vi "App - analyze RUS V6.vi"() -> ()   [LabVIEW 2015] (continued)
path"=path "D:/Data/Ultrasound/LSCO/LSCO22__130814c/5_Cooling_2nd_try/September_2014/091614/137.30000K_500_2500_2.10000V_0.00000T_Sep16-2014__18-33-45_001_091614.bin", "last mod"=timestamp(3493751625 s since 1904-01-01), "file name str"="D:\\Data\\Ultrasound\\LSCO\\LSCO22__130814c\\5_Cooling_2nd_try\\September_2014\\091614\\137.30000K_500_2500_2.10000V_0.00000T_Sep16-2014__18-33-45_001_091614.bin", "mod time(min)"=58229193.75, "file format"=enum."binary", "power(V)"=2.1, "Magn Field(T) "=0.0}, {"temperature"=137.004, "temperature str"="137.00400", "file path"=path "D:/Data/Ultrasound/LSCO/LSCO22__130814c/5_Cooling_2nd_try/September_2014/091614/137.00400K_500_2500_2.10000V_0.00000T_Sep16-2014__18-35-05_001_091614.bin", "last mod"=timestamp(3493751705 s since 1904-01-01), "file name str"="D:\\Data\\Ultrasound\\LSCO\\LSCO22__130814c\\5_Cooling_2nd_try\\September_2014\\091614\\137.00400K_500_2500_2.10000V_0.00000T_Sep16-2014__18-35-05_001_091614.bin", "mod time(min)"=58229195.083333336, "file format"=enum."binary", "power(V)"=2.1, "Magn Field(T) "=0.0}, {"temperature"=136.689, "temperature str"="136.68900", "file path"=path "D:/Data/Ultrasound/LSCO/LSCO22__130814c/5_Cooling_2nd_try/September_2014/091614/136.68900K_500_2500_2.10000V_0.00000T_Sep16-2014__18-36-24_001_091614.bin", "last mod"=timestamp(3493751784 s since 1904-01-01), "file name str"="D:\\Data\\Ultrasound\\LSCO\\LSCO22__130814c\\5_Cooling_2nd_try\\September_2014\\091614\\136.68900K_500_2500_2.10000V_0.00000T_Sep16-2014__18-36-24_001_091614.bin", "mod time(min)"=58229196.4, "file format"=enum."binary", "power(V)"=2.1, "Magn Field(T) "=0.0}, {"temperature"=136.379, "temperature str"="136.37900", "file path"=path "D:/Data/Ultrasound/LSCO/LSCO22__130814c/5_Cooling_2nd_try/September_2014/091614/136.37900K_500_2500_2.10000V_0.00000T_Sep16-2014__18-37-44_001_091614.bin", "last mod"=timestamp(3493751864 s since 1904-01-01), "file name str"="D:\\Data\\Ultrasound\\LSCO\\LSCO22__130814c\\5_Cooling_2nd_try\\September_2014\\091614\\136.37900K_500_2500_2.10000V_0.00000T_Sep16-2014__18-37-44_001_091614.bin", "mod time(min)"=58229197.733333334, "file format"=enum."binary", "power(V)"=2.1, "Magn Field(T) "=0.0}, {"temperature"=136.08, "temperature str"="136.08000", "file path"=path "D:/Data/Ultrasound/LSCO/LSCO22__130814c/5_Cooling_2nd_try/September_2014/091614/136.08000K_500_2500_2.10000V_0.00000T_Sep16-2014__18-39-03_001_091614.bin", "last mod"=timestamp(3493751943 s since 1904-01-01), "file name str"="D:\\Data\\Ultrasound\\LSCO\\LSCO22__130814c\\5_Cooling_2nd_try\\September_2014\\091614\\136.08000K_500_2500_2.10000V_0.00000T_Sep16-2014__18-39-03_001_091614.bin", "mod time(min)"=58229199.05, "file format"=enum."binary", "power(V)"=2.1, "Magn Field(T) "=0.0}, {"temperature"=135.77, "temperature str"="135.77000", "file path"=path "D:/Data/Ultrasound/LSCO/LSCO22__130814c/5_Cooling_2nd_try/September_2014/091614/135.77000K_500_2500_2.10000V_0.00000T_Sep16-2014__18-40-22_001_091614.bin", "last mod"=timestamp(3493752022 s since 1904-01-01), "file name str"="D:\\Data\\Ultrasound\\LSCO\\LSCO22__130814c\\5_Cooling_2nd_try\\September_2014\\091614\\135.77000K_500_2500_2.10000V_0.00000T_Sep16-2014__18-40-22_001_091614.bin", "mod time(min)"=58229200.36666667, "file format"=enum."binary", "power(V)"=2.1, "Magn Field(T) "=0.0}, {"temperature"=135.475, "temperature str"="135.47500", "file path"=path "D:/Data/Ultrasound/LSCO/LSCO22__130814c/5_Cooling_2nd_try/September_2014/091614/135.47500K_500_2500_2.10000V_0.00000T_Sep16-2014__18-41-42_001_091614.bin", "last mod"=timestamp(3493752102 s since 1904-01-01), "file name str"="D:\\Data\\Ultrasound\\LSCO\\LSCO22__130814c\\5_Cooling_2nd_try\\September_2014\\091614\\135.47500K_500_2500_2.10000V_0.00000T_Sep16-2014__18-41-42_001_091614.bin", "mod time(min)"=58229201.7, "file format"=enum."binary", "power(V)"=2.1, "Magn Field(T) "=0.0}, {"temperature"=135.167, "temperature str"="135.16700", "file path"=path "D:/Data/Ultrasound/LSCO/LSCO22__130814c/5_Cooling_2nd_try/September_2014/091614/135.16700K_500_2500_2.10000V_0.00000T_Sep16-2014__18-43-01_001_091614.bin", "last mod"=timestamp(3493752181 s since 1904-01-01), "file name str"="D:\\Data\\Ultrasound\\LSCO\\LSCO22__130814c\\5_Cooling_2nd_try\\September_2014\\091614\\135.16700K_500_2500_2.10000V_0.00000T_Sep16-2014__18-43-01_001_091614.bin", "mod time(min)"=58229203.016666666, "file format"=enum."binary", "power(V)"=2.1, "Magn Field(T) "=0.0}, {"temperature"=134.859, "temperature str"="134.85900", "file path"=path "D:/Data/Ultrasound/LSCO/LSCO22__130814c/5_Cooling_2nd_try/September_2014/091614/134.85900K_500_2500_2.10000V_0.00000T_Sep16-2014__18-44-20_001_091614.bin", "last mod"=timestamp(3493752260 s since 1904-01-01), "file name str"="D:\\Data\\Ultrasound\\LSCO\\LSCO22__130814c\\5_Cooling_2nd_try\\September_2014\\091614\\134.85900K_500_2500_2.10000V_0.00000T_Sep16-2014__18-44-20_001_091614.bin", "mod time(min)"=58229204.333333336, "file format"=enum."binary", "power(V)"=2.1, "Magn Field(T) "=0.0}, {"temperature"=134.565, "temperature str"="134.56500", "file path"=path "D:/Data/Ultrasound/LSCO/LSCO22__130814c/5_Cooling_2nd_try/September_2014/091614/134.56500K_500_2500_2.10000V_0.00000T_Sep16-2014__18-45-40_001_091614.bin", "last mod"=timestamp(3493752340 s since 1904-01-01), "file name str"="D:\\Data\\Ultrasound\\LSCO\\LSCO22__130814c\\5_Cooling_2nd_try\\September_2014\\091614\\134.56500K_500_2500_2.10000V_0.00000T_Sep16-2014__18-45-40_001_091614.bin", "mod time(min)"=58229205.666666664, "file format"=enum."binary", "power(V)"=2.1, "Magn Field(T) "=0.0}, {"temperature"=134.259, "temperature str"="134.25900", "file path"=path "D:/Data/Ultrasound/LSCO/LSCO22__130814c/5_Cooling_2nd_try/September_2014/091614/134.25900K_500_2500_2.10000V_0.00000T_Sep16-2014__18-46-59_001_091614.bin", "last mod"=timestamp(3493752419 s since 1904-01-01), "file name str"="D:\\Data\\Ultrasound\\LSCO\\LSCO22__130814c\\5_Cooling_2nd_try\\September_2014\\091614\\134.25900K_500_2500_2.10000V_0.00000T_Sep16-2014__18-46-59_001_091614.bin", "mod time(min)"=58229206.983333334, "file format"=enum."binary", "power(V)"=2.1, "Magn Field(T) "=0.0}, {"temperature"=133.967, "temperature str"="133.96700", "file path"=path "D:/Data/Ultrasound/LSCO/LSCO22__130814c/5_Cooling_2nd_try/September_2014/091614/133.96700K_500_2500_2.10000V_0.00000T_Sep16-2014__18-48-19_001_091614.bin", "last mod"=timestamp(3493752499 s since 1904-01-01), "file name str"="D:\\Data\\Ultrasound\\LSCO\\LSCO22__130814c\\5_Cooling_2nd_try\\September_2014\\091614\\133.96700K_500_2500_2.10000V_0.00000T_Sep16-2014__18-48-19_001_091614.bin", "mod time(min)"=58229208.31666667, "file format"=enum."binary", "power(V)"=2.1, "Magn Field(T) "=0.0}, {"temperature"=133.655, "temperature str"="133.65500", "file path"=path "D:/Data/Ultrasound/LSCO/LSCO22__130814c/5_Cooling_2nd_try/September_2014/091614/133.65500K_500_2500_2.10000V_0.00000T_Sep16-2014__18-49-38_001_091614.bin", "last mod"=timestamp(3493752578 s since 1904-01-01), "file name str"="D:\\Data\\Ultrasound\\LSCO\\LSCO22__130814c\\5_Cooling_2nd_try\\September_2014\\091614\\133.65500K_500_2500_2.10000V_0.00000T_Sep16-2014__18-49-38_001_091614.bin", "mod time(min)"=58229209.63333333, "file format"=enum."binary", "power(V)"=2.1, "Magn Field(T) "=0.0}, {"temperature"=133.359, "temperature str"="133.35900", "file path"=path "D:/Data/Ultrasound/LSCO/LSCO22__130814c/5_Cooling_2nd_try/September_2014/091614/133.35900K_500_2500_2.10000V_0.00000T_Sep16-2014__18-50-57_001_091614.bin", "last mod"=timestamp(3493752657 s since 1904-01-01), "file name str"="D:\\Data\\Ultrasound\\LSCO\\LSCO22__130814c\\5_Cooling_2nd_try\\September_2014\\091614\\133.35900K_500_2500_2.10000V_0.00000T_Sep16-2014__18-50-57_001_091614.bin", "mod time(min)"=58229210.95, "file format"=enum."binary", "power(V)"=2.1, "Magn Field(T) "=0.0}, {"temperature"=133.076, "temperature str"="133.07600", "file path"=path "D:/Data/Ultrasound/LSCO/LSCO22__130814c/5_Cooling_2nd_try/September_2014/091614/133.07600K_500_2500_2.10000V_0.00000T_Sep16-2014__18-52-17_001_091614.bin", "last mod"=timestamp(3493752737 s since 1904-01-01), "file name str"="D:\\Data\\Ultrasound\\LSCO\\LSCO22__130814c\\5_Cooling_2nd_try\\September_2014\\091614\\133.07600K_500_2500_2.10000V_0.00000T_Sep16-2014__18-52-17_001_091614.bin", "mod time(min)"=58229212.28333333, "file format"=enum."binary", "power(V)"=2.1, "Magn Field(T) "=0.0}, {"temperature"=132.767, "temperature str"="132.76700", "file path"=path "D:/Data/Ultrasound/LSCO/LSCO22__130814c/5_Cooling_2nd_try/September_2014/091614/132.76700K_500_2500_2.10000V_0.00000T_Sep16-2014__18-53-36_001_091614.bin", "last mod"=timestamp(3493752816 s since 1904-01-01), "file name str"="D:\\Data\\Ultrasound\\LSCO\\LSCO22__130814c\\5_Cooling_2nd_try\\September_2014\\091614\\132.76700K_500_2500_2.10000V_0.00000T_Sep16-2014__18-53-36_001_091614.bin", "mod time(min)"=58229213.6, "file format"=enum."binary", "power(V)"=2.1, "Magn Field(T) "=0.0}, {"temperature"=132.465, "temperature str"="132.46500", "file path"=path "D:/Data/Ultrasound/LSCO/LSCO22__130814c/5_Cooling_2nd_try/September_2014/091614/132.46500K_500_2500_2.10000V_0.00000T_Sep16-2014__18-54-56_001_091614.bin", "last mod"=timestamp(3493752896 s since 1904-01-01), "file name str"="D:\\Data\\Ultrasound\\LSCO\\LSCO22__130814c\\5_Cooling_2nd_try\\September_2014\\091614\\132.46500K_500_2500_2.10000V_0.00000T_Sep16-2014__18-54-56_001_091614.bin", "mod time(min)"=58229214.93333333, "file format"=enum."binary", "power(V)"=2.1, "Magn Field(T) "=0.0}, {"temperature"=132.185, "temperature str"="132.18500", "file path"=path "D:/Data/Ultrasound/LSCO/LSCO22__130814c/5_Cooling_2nd_try/September_2014/091614/132.18500K_500_2500_2.10000V_0.00000T_Sep16-2014__18-56-15_001_091614.bin", "last mod"=timestamp(3493752975 s since 1904-01-01), "file name str"="D:\\Data\\Ultrasound\\LSCO\\LSCO22__130814c\\5_Cooling_2nd_try\\September_2014\\091614\\132.18500K_500_2500_2.10000V_0.00000T_Sep16-2014__18-56-15_001_091614.bin", "mod time(min)"=58229216.25, "file format"=enum."binary", "power(V)"=2.1, "Magn Field(T) "=0.0}, {"temperature"=131.882, "temperature str"="131.88200", "file path"=path "D:/Data/Ultrasound/LSCO/LSCO22__130814c/5_Cooling_2nd_try/September_2014/091614/131.88200K_500_2500_2.10000V_0.00000T_Sep16-2014__18-57-34_001_091614.bin", "last mod"=timestamp(3493753054 s since 1904-01-01), "file name str"="D:\\Data\\Ultrasound\\LSCO\\LSCO22__130814c\\5_Cooling_2nd_try\\September_2014\\091614\\131.88200K_500_2500_2.10000V_0.00000T_Sep16-2014__18-57-34_001_091614.bin", "mod time(min)"=58229217.56666667, "file format"=enum."binary", "power(V)"=2.1, "Magn Field(T) "=0.0}, {"temperature"=131.592, "temperature str"="131.59200", "file path"=path "D:/Data/Ultrasound/LSCO/LSCO22__130814c/5_Cooling_2nd_try/September_2014/091614/131.59200K_500_2500_2.10000V_0.00000T_Sep16-2014__18-58-54_001_091614.bin", "last mod"=timestamp(3493753134 s since 1904-01-01), "file name str"="D:\\Data\\Ultrasound\\LSCO\\LSCO22__130814c\\5_Cooling_2nd_try\\September_2014\\091614\\131.59200K_500_2500_2.10000V_0.00000T_Sep16-2014__18-58-54_001_091614.bin", "mod time(min)"=58229218.9, "file format"=enum."binary", "power(V)"=2.1, "Magn Field(T) "=0.0}, {"temperature"=131.299, "temperature str"="131.29900", "file path"=path "D:/Data/Ultrasound/LSCO/LSCO22__130814c/5_Cooling_2nd_try/September_2014/091614/131.29900K_500_2500_2.10000V_0.00000T_Sep16-2014__19-00-13_001_091614.bin", "last mod"=timestamp(3493753213 s since 1904-01-01), "file name str"="D:\\Data\\Ultrasound\\LSCO\\LSCO22__130814c\\5_Cooling_2nd_try\\September_2014\\091614\\131.29900K_500_2500_2.10000V_0.00000T_Sep16-2014__19-00-13_001_091614.bin", "mod time(min)"=58229220.21666667, "file format"=enum."binary", "power(V)"=2.1, "Magn Field(T) "=0.0}, {"temperature"=131.007, "temperature str"="131.00700", "file path"=path "D:/Data/Ultrasound/LSCO/LSCO22__130814c/5_Cooling_2nd_try/September_2014/091614/131.00700K_500_2500_2.10000V_0.00000T_Sep16-2014__19-01-32_001_091614.bin", "last mod"=timestamp(3493753292 s since 1904-01-01), "file name str"="D:\\Data\\Ultrasound\\LSCO\\LSCO22__130814c\\5_Cooling_2nd_try\\September_2014\\091614\\131.00700K_500_2500_2.10000V_0.00000T_Sep16-2014__19-01-32_001_091614.bin", "mod time(min)"=58229221.53333333, "file format"=enum."binary", "power(V)"=2.1, "Magn Field(T) "=0.0}, {"temperature"=130.718, "temperature str"="130.71800", "file path"=path "D:/Data/Ultrasound/LSCO/LSCO22__130814c/5_Cooling_2nd_try/September_2014/091614/130.71800K_500_2500_2.10000V_0.00000T_Sep16-2014__19-02-52_001_091614.bin", "last mod"=timestamp(3493753372 s since 1904-01-01), "file name str"="D:\\Data\\Ultrasound\\LSCO\\LSCO22__130814c\\5_Cooling_2nd_try\\September_2014\\091614\\130.71800K_500_2500_2.10000V_0.00000T_Sep16-2014__19-02-52_001_091614.bin", "mod time(min)"=58229222.86666667, "file format"=enum."binary", "power(V)"=2.1, "Magn Field(T) "=0.0}, {"temperature"=130.427, "temperature str"="130.42700", "file path"=path "D:/Data/Ultrasound/LSCO/LSCO22__130814c/5_Cooling_2nd_try/September_2014/091614/130.42700K_500_2500_2.10000V_0.00000T_Sep16-2014__19-04-11_001_091614.bin", "last mod"=timestamp(3493753451 s since 1904-01-01), "file name str"="D:\\Data\\Ultrasound\\LSCO\\LSCO22__130814c\\5_Cooling_2nd_try\\September_2014\\091614\\130.42700K_500_2500_2.10000V_0.00000T_Sep16-2014__19-04-11_001_091614.bin", "mod time(min)"=58229224.18333333, "file format"=enum."binary", "power(V)"=2.1, "Magn Field(T) "=0.0}, {"temperature"=130.147, "temperature str"="130.14700", "file path"=path "D:/Data/Ultrasound/LSCO/LSCO22__130814c/5_Cooling_2nd_try/September_2014/091614/130.14700K_500_2500_2.10000V_0.00000T_Sep16-2014__19-05-31_001_091614.bin", "last mod"=timestamp(3493753531 s since 1904-01-01), "file name str"="D:\\Data\\Ultrasound\\LSCO\\LSCO22__130814c\\5_Cooling_2nd_try\\September_2014\\091614\\130.14700K_500_2500_2.10000V_0.00000T_Sep16-2014__19-05-31_001_091614.bin", "mod time(min)"=58229225.516666666, "file format"=enum."binary", "power(V)"=2.1, "Magn Field(T) "=0.0}, {"temperature"=129.849, "temperature str"="129.84900", "file path"=path "D:/Data/Ultrasound/LSCO/LSCO22__130814c/5_Cooling_2nd_try/September_2014/091614/129.84900K_500_2500_2.10000V_0.00000T_Sep16-2014__19-06-50_001_091614.bin", "last mod"=timestamp(3493753610 s since 1904-01-01), "file name str"="D:\\Data\\Ultrasound\\LSCO\\LSCO22__130814c\\5_Cooling_2nd_try\\September_2014\\091614\\129.84900K_500_2500_2.10000V_0.00000T_Sep16-2014__19-06-50_001_091614.bin", "mod time(min)"=58229226.833333336, "file format"=enum."binary", "power(V)"=2.1, "Magn Field(T) "=0.0}, {"temperature"=129.561, "temperature str"="129.56100", "file path"=path "D:/Data/Ultrasound/LSCO/LSCO22__130814c/5_Cooling_2nd_try/September_2014/091614/129.56100K_500_2500_2.10000V_0.00000T_Sep16-2014__19-08-09_001_091614.bin", "last mod"=timestamp(3493753689 s since 1904-01-01), "file name str"="D:\\Data\\Ultrasound\\LSCO\\LSCO22__130814c\\5_Cooling_2nd_try\\September_2014\\091614\\129.56100K_500_2500_2.10000V_0.00000T_Sep16-2014__19-08-09_001_091614.bin", "mod time(min)"=58229228.15, "file format"=enum."binary", "power(V)"=2.1, "Magn Field(T) "=0.0}, {"temperature"=129.282, "temperature str"="129.28200", "file path"=path "D:/Data/Ultrasound/LSCO/LSCO22__130814c/5_Cooling_2nd_try/September_2014/091614/129.28200K_500_2500_2.10000V_0.00000T_Sep16-2014__19-09-29_001_091614.bin", "last mod"=timestamp(3493753769 s since 1904-01-01), "file name str"="D:\\Data\\Ultrasound\\LSCO\\LSCO22__130814c\\5_Cooling_2nd_try\\September_2014\\091614\\129.28200K_500_2500_2.10000V_0.00000T_Sep16-2014__19-09-29_001_091614.bin", "mod time(min)"=58229229.483333334, "file format"=enum."binary", "power(V)"=2.1, "Magn Field(T) "=0.0}, {"temperature"=128.991, "temperature str"="128.99100", "file path"=path "D:/Data/Ultrasound/LSCO/LSCO22__130814c/5_Cooling_2nd_try/September_2014/091614/128.99100K_500_2500_2.10000V_0.00000T_Sep16-2014__19-10-48_001_091614.bin", "last mod"=timestamp(3493753848 s since 1904-01-01), "file name str"="D:\\Data\\Ultrasound\\LSCO\\LSCO22__130814c\\5_Cooling_2nd_try\\September_2014\\091614\\128.99100K_500_2500_2.10000V_0.00000T_Sep16-2014__19-10-48_001_091614.bin", "mod time(min)"=58229230.8, "file format"=enum."binary", "power(V)"=2.1, "Magn Field(T) "=0.0}, {"temperature"=128.717, "temperature str"="128.71700", "file path"=path "D:/Data/Ultrasound/LSCO/LSCO22__130814c/5_Cooling_2nd_try/September_2014/091614/128.71700K_500_2500_2.10000V_0.00000T_Sep16-2014__19-12-07_001_091614.bin", "last mod"=timestamp(3493753927 s since 1904-01-01), "file name str"="D:\\Data\\Ultrasound\\LSCO\\LSCO22__130814c\\5_Cooling_2nd_try\\September_2014\\091614\\128.71700K_500_2500_2.10000V_0.00000T_Sep16-2014__19-12-07_001_091614.bin", "mod time(min)"=58229232.11666667, "file format"=enum."binary", "power(V)"=2.1, "Magn Field(T) "=0.0}, {"temperature"=128.421, "temperature str"="128.42100", "file path"=path "D:/Data/Ultrasound/LSCO/LSCO22__130814c/5_Cooling_2nd_try/September_2014/091614/128.42100K_500_2500_2.10000V_0.00000T_Sep16-2014__19-13-27_001_091614.bin", "last mod"=timestamp(3493754007 s since 1904-01-01), "file name str"="D:\\Data\\Ultrasound\\LSCO\\LSCO22__130814c\\5_Cooling_2nd_try\\September_2014\\091614\\128.42100K_500_2500_2.10000V_0.00000T_Sep16-2014__19-13-27_001_091614.bin", "mod time(min)"=58229233.45, "file format"=enum."binary", "power(V)"=2.1, "Magn Field(T) "=0.0}, {"temperature"=128.135, "temperature str"="128.13500", "file path"=path "D:/Data/Ultrasound/LSCO/LSCO22__130814c/5_Cooling_2nd_try/September_2014/091614/128.13500K_500_2500_2.10000V_0.00000T_Sep16-2014__19-14-46_001_091614.bin", "last mod"=timestamp(3493754086 s since 1904-01-01), "file name str"="D:\\Data\\Ultrasound\\LSCO\\LSCO22__130814c\\5_Cooling_2nd_try\\September_2014\\091614\\128.13500K_500_2500_2.10000V_0.00000T_Sep16-2014__19-14-46_001_091614.bin", "mod time(min)"=58229234.766666666, "file format"=enum."binary", "power(V)"=2.1, "Magn Field(T) "=0.0}, {"temperature"=127.874, "temperature str"="127.87400", "file path"=path "D:/Data/Ultrasound/LSCO/LSCO22__130814c/5_Cooling_2nd_try/September_2014/091614/127.87400K_500_2500_2.10000V_0.00000T_Sep16-2014__19-16-06_001_091614.bin", "last mod"=timestamp(3493754166 s since 1904-01-01), "file name str"="D:\\Data\\Ultrasound\\LSCO\\LSCO22__130814c\\5_Cooling_2nd_try\\September_2014\\091614\\127.87400K_500_2500_2.10000V_0.00000T_Sep16-2014__19-16-06_001_091614.bin", "mod time(min)"=58229236.1, "file format"=enum."binary", "power(V)"=2.1, "Magn Field(T) "=0.0}, {"temperature"=127.58, "temperature str"="127.58000", "file path"=path "D:/Data/Ultrasound/LSCO/LSCO22__130814c/5_Cooling_2nd_try/September_2014/091614/127.58000K_500_2500_2.10000V_0.00000T_Sep16-2014__19-17-25_001_091614.bin", "last mod"=timestamp(3493754245 s since 1904-01-01), "file name str"="D:\\Data\\Ultrasound\\LSCO\\LSCO22__130814c\\5_Cooling_2nd_try\\September_2014\\091614\\127.58000K_500_2500_2.10000V_0.00000T_Sep16-2014__19-17-25_001_091614.bin", "mod time(min)"=58229237.416666664, "file format"=enum."binary", "power(V)"=2.1, "Magn Field(T) "=0.0}, {"temperature"=127.303, "temperature str"="127.30300", "file path"=path "D:/Data/Ultrasound/LSCO/LSCO22__130814c/5_Cooling_2nd_try/September_2014/091614/127.30300K_500_2500_2.10000V_0.00000T_Sep16-2014__19-18-44_001_091614.bin", "last mod"=timestamp(3493754324 s since 1904-01-01), "file name str"="D:\\Data\\Ultrasound\\LSCO\\LSCO22__130814c\\5_Cooling_2nd_try\\September_2014\\091614\\127.30300K_500_2500_2.10000V_0.00000T_Sep16-2014__19-18-44_001_091614.bin", "mod time(min)"=58229238.733333334, "file format"=enum."binary", "power(V)"=2.1, "Magn Field(T) "=0.0}, {"temperature"=127.032, "temperature str"="127.03200", "file path"=path "D:/Data/Ultrasound/LSCO/LSCO22__130814c/5_Cooling_2nd_try/September_2014/091614/127.03200K_500_2500_2.10000V_0.00000T_Sep16-2014__19-20-04_001_091614.bin", "last mod"=timestamp(3493754404 s since 1904-01-01), "file name str"="D:\\Data\\Ultrasound\\LSCO\\LSCO22__130814c\\5_Cooling_2nd_try\\September_2014\\091614\\127.03200K_500_2500_2.10000V_0.00000T_Sep16-2014__19-20-04_001_091614.bin", "mod time(min)"=58229240.06666667, "file format"=enum."binary", "power(V)"=2.1, "Magn Field(T) "=0.0}, {"temperature"=126.745, "temperature str"="126.74500", "file path"=path "D:/Data/Ultrasound/LSCO/LSCO22__130814c/5_Cooling_2nd_try/September_2014/091614/126.74500K_500_2500_2.10000V_0.00000T_Sep16-2014__19-21-23_001_091614.bin", "last mod"=timestamp(3493754483 s since 1904-01-01), "file name str"="D:\\Data\\Ultrasound\\LSCO\\LSCO22__130814c\\5_Cooling_2nd_try\\September_2014\\091614\\126.74500K_500_2500_2.10000V_0.00000T_Sep16-2014__19-21-23_001_091614.bin", "mod time(min)"=58229241.38333333, "file format"=enum."binary", "power(V)"=2.1, "Magn Field(T) "=0.0}, {"temperature"=126.472, "temperature str"="126.47200", "file path"=path "D:/Data/Ultrasound/LSCO/LSCO22__130814c/5_Cooling_2nd_try/September_2014/091614/126.47200K_500_2500_2.10000V_0.00000T_Sep16-2014__19-22-43_001_091614.bin", "last mod"=timestamp(3493754563 s since 1904-01-01), "file name str"="D:\\Data\\Ultrasound\\LSCO\\LSCO22__130814c\\5_Cooling_2nd_try\\September_2014\\091614\\126.47200K_500_2500_2.10000V_0.00000T_Sep16-2014__19-22-43_001_091614.bin", "mod time(min)"=58229242.71666667, "file format"=enum."binary", "power(V)"=2.1, "Magn Field(T) "=0.0}, {"temperature"=126.195, "temperature str"="126.19500", "file path"=path "D:/Data/Ultrasound/LSCO/LSCO22__130814c/5_Cooling_2nd_try/September_2014/091614/126.19500K_500_2500_2.10000V_0.00000T_Sep16-2014__19-24-02_001_091614.bin", "last mod"=timestamp(3493754642 s since 1904-01-01), "file name str"="D:\\Data\\Ultrasound\\LSCO\\LSCO22__130814c\\5_Cooling_2nd_try\\September_2014\\091614\\126.19500K_500_2500_2.10000V_0.00000T_Sep16-2014__19-24-02_001_091614.bin", "mod time(min)"=58229244.03333333, "file format"=enum."binary", "power(V)"=2.1, "Magn Field(T) "=0.0}, {"temperature"=125.926, "temperature str"="125.92600", "file path"=path "D:/Data/Ultrasound/LSCO/LSCO22__130814c/5_Cooling_2nd_try/September_2014/091614/125.92600K_500_2500_2.10000V_0.00000T_Sep16-2014__19-25-21_001_091614.bin", "last mod"=timestamp(3493754721 s since 1904-01-01), "file name str"="D:\\Data\\Ultrasound\\LSCO\\LSCO22__130814c\\5_Cooling_2nd_try\\September_2014\\091614\\125.92600K_500_2500_2.10000V_0.00000T_Sep16-2014__19-25-21_001_091614.bin", "mod time(min)"=58229245.35, "file format"=enum."binary", "power(V)"=2.1, "Magn Field(T) "=0.0}, {"temperature"=125.648, "temperature str"="125.64800", "file path"=path "D:/Data/Ultrasound/LSCO/LSCO22__130814c/5_Cooling_2nd_try/September_2014/091614/125.64800K_500_2500_2.10000V_0.00000T_Sep16-2014__19-26-41_001_091614.bin", "last mod"=timestamp(3493754801 s since 1904-01-01), "file name str"="D:\\Data\\Ultrasound\\LSCO\\LSCO22__130814c\\5_Cooling_2nd_try\\September_2014\\091614\\125.64800K_500_2500_2.10000V_0.00000T_Sep16-2014__19-26-41_001_091614.bin", "mod time(min)"=58229246.68333333, "file format"=enum."binary", "power(V)"=2.1, "Magn Field(T) "=0.0}, {"temperature"=125.371, "temperature str"="125.37100", "file path"=path "D:/Data/Ultrasound/LSCO/LSCO22__130814c/5_Cooling_2nd_try/September_2014/091614/125.37100K_500_2500_2.10000V_0.00000T_Sep16-2014__19-28-00_001_091614.bin", "last mod"=timestamp(3493754880 s since 1904-01-01), "file name str"="D:\\Data\\Ultrasound\\LSCO\\LSCO22__130814c\\5_Cooling_2nd_try\\September_2014\\091614\\125.37100K_500_2500_2.10000V_0.00000T_Sep16-2014__19-28-00_001_091614.bin", "mod time(min)"=58229248.0, "file format"=enum."binary", "power(V)"=2.1, "Magn Field(T) "=0.0}, {"temperature"=125.102, "temperature str"="125.10200", "file path"=path "D:/Data/Ultrasound/LSCO/LSCO22__130814c/5_Cooling_2nd_try/September_2014/091614/125.10200K_500_2500_2.10000V_0.00000T_Sep16-2014__19-29-19_001_091614.bin", "last mod"=timestamp(3493754959 s since 1904-01-01), "file name str"="D:\\Data\\Ultrasound\\LSCO\\LSCO22__130814c\\5_Cooling_2nd_try\\September_2014\\091614\\125.10200K_500_2500_2.10000V_0.00000T_Sep16-2014__19-29-19_001_091614.bin", "mod time(min)"=58229249.31666667, "file format"=enum."binary", "power(V)"=2.1, "Magn Field(T) "=0.0}, {"temperature"=124.83, "temperature str"="124.83000", "file path"=path "D:/Data/Ultrasound/LSCO/LSCO22__130814c/5_Cooling_2nd_try/September_2014/091614/124.83000K_500_2500_2.10000V_0.00000T_Sep16-2014__19-30-39_001_091614.bin", "last mod"=timestamp(3493755039 s since 1904-01-01), "file name str"="D:\\Data\\Ultrasound\\LSCO\\LSCO22__130814c\\5_Cooling_2nd_try\\September_2014\\091614\\124.83000K_500_2500_2.10000V_0.00000T_Sep16-2014__19-30-39_001_091614.bin", "mod time(min)"=58229250.65, "file format"=enum."binary", "power(V)"=2.1, "Magn Field(T) "=0.0}, {"temperature"=124.565, "temperature str"="124.56500", "file path"=path "D:/Data/Ultrasound/LSCO/LSCO22__130814c/5_Cooling_2nd_try/September_2014/091614/124.56500K_500_2500_2.10000V_0.00000T_Sep16-2014__19-31-58_001_091614.bin", "last mod"=timestamp(3493755118 s since 1904-01-01), "file name str"="D:\\Data\\Ultrasound\\LSCO\\LSCO22__130814c\\5_Cooling_2nd_try\\September_2014\\091614\\124.56500K_500_2500_2.10000V_0.00000T_Sep16-2014__19-31-58_001_091614.bin", "mod time(min)"=58229251.96666667, "file format"=enum."binary", "power(V)"=2.1, "Magn Field(T) "=0.0}, {"temperature"=124.29, "temperature str"="124.29000", "file path"=path "D:/Data/Ultrasound/LSCO/LSCO22__130814c/5_Cooling_2nd_try/September_2014/091614/124.29000K_500_2500_2.10000V_0.00000T_Sep16-2014__19-33-18_001_091614.bin", "last mod"=timestamp(3493755198 s since 1904-01-01), "file name str"="D:\\Data\\Ultrasound\\LSCO\\LSCO22__130814c\\5_Cooling_2nd_try\\September_2014\\091614\\124.29000K_500_2500_2.10000V_0.00000T_Sep16-2014__19-33-18_001_091614.bin", "mod time(min)"=58229253.3, "file format"=enum."binary", "power(V)"=2.1, "Magn Field(T) "=0.0}, {"temperature"=124.019, "temperature str"="124.01900", "file path"=path "D:/Data/Ultrasound/LSCO/LSCO22__130814c/5_Cooling_2nd_try/September_2014/091614/124.01900K_500_2500_2.10000V_0.00000T_Sep16-2014__19-34-37_001_091614.bin", "last mod"=timestamp(3493755277 s since 1904-01-01), "file name str"="D:\\Data\\Ultrasound\\LSCO\\LSCO22__130814c\\5_Cooling_2nd_try\\September_2014\\091614\\124.01900K_500_2500_2.10000V_0.00000T_Sep16-2014__19-34-37_001_091614.bin", "mod time(min)"=58229254.61666667, "file format"=enum."binary", "power(V)"=2.1, "Magn Field(T) "=0.0}, {"temperature"=123.76, "temperature str"="123.76000", "file path"=path "D:/Data/Ultrasound/LSCO/LSCO22__130814c/5_Cooling_2nd_try/September_2014/091614/123.76000K_500_2500_2.10000V_0.00000T_Sep16-2014__19-35-56_001_091614.bin", "last mod"=timestamp(3493755356 s since 1904-01-01), "file name str"="D:\\Data\\Ultrasound\\LSCO\\LSCO22__130814c\\5_Cooling_2nd_try\\September_2014\\091614\\123.76000K_500_2500_2.10000V_0.00000T_Sep16-2014__19-35-56_001_091614.bin", "mod time(min)"=58229255.93333333, "file format"=enum."binary", "power(V)"=2.1, "Magn Field(T) "=0.0}, {"temperature"=123.485, "temperature str"="123.48500", "file path"=path "D:/Data/Ultrasound/LSCO/LSCO22__130814c/5_Cooling_2nd_try/September_2014/091614/123.48500K_500_2500_2.10000V_0.00000T_Sep16-2014__19-37-16_001_091614.bin", "last mod"=timestamp(3493755436 s since 1904-01-01), "file name str"="D:\\Data\\Ultrasound\\LSCO\\LSCO22__130814c\\5_Cooling_2nd_try\\September_2014\\091614\\123.48500K_500_2500_2.10000V_0.00000T_Sep16-2014__19-37-16_001_091614.bin", "mod time(min)"=58229257.266666666, "file format"=enum."binary", "power(V)"=2.1, "Magn Field(T) "=0.0}, {"temperature"=123.221, "temperature str"="123.22100", "file path"=path "D:/Data/Ultrasound/LSCO/LSCO22__130814c/5_Cooling_2nd_try/September_2014/091614/123.22100K_500_2500_2.10000V_0.00000T_Sep16-2014__19-38-35_001_091614.bin", "last mod"=timestamp(3493755515 s since 1904-01-01), "file name str"="D:\\Data\\Ultrasound\\LSCO\\LSCO22__130814c\\5_Cooling_2nd_try\\September_2014\\091614\\123.22100K_500_2500_2.10000V_0.00000T_Sep16-2014__19-38-35_001_091614.bin", "mod time(min)"=58229258.583333336, "file format"=enum."binary", "power(V)"=2.1, "Magn Field(T) "=0.0}, {"temperature"=122.957, "temperature str"="122.95700", "file path"=path "D:/Data/Ultrasound/LSCO/LSCO22__130814c/5_Cooling_2nd_try/September_2014/091614/122.95700K_500_2500_2.10000V_0.00000T_Sep16-2014__19-39-54_001_091614.bin", "last mod"=timestamp(3493755594 s since 1904-01-01), "file name str"="D:\\Data\\Ultrasound\\LSCO\\LSCO22__130814c\\5_Cooling_2nd_try\\September_2014\\091614\\122.95700K_500_2500_2.10000V_0.00000T_Sep16-2014__19-39-54_001_091614.bin", "mod time(min)"=58229259.9, "file format"=enum."binary", "power(V)"=2.1, "Magn Field(T) "=0.0}, {"temperature"=122.69, "temperature str"="122.69000", "file path"=path "D:/Data/Ultrasound/LSCO/LSCO22__130814c/5_Cooling_2nd_try/September_2014/091614/122.69000K_500_2500_2.10000V_0.00000T_Sep16-2014__19-41-14_001_091614.bin", "last mod"=timestamp(3493755674 s since 1904-01-01), "file name str"="D:\\Data\\Ultrasound\\LSCO\\LSCO22__130814c\\5_Cooling_2nd_try\\September_2014\\091614\\122.69000K_500_2500_2.10000V_0.00000T_Sep16-2014__19-41-14_001_091614.bin", "mod time(min)"=58229261.233333334, "file format"=enum."binary", "power(V)"=2.1, "Magn Field(T) "=0.0}, {"temperature"=122.431, "temperature str"="122.43100", "file path"=path "D:/Data/Ultrasound/LSCO/LSCO22__130814c/5_Cooling_2nd_try/September_2014/091614/122.43100K_500_2500_2.10000V_0.00000T_Sep16-2014__19-42-33_001_091614.bin", "last mod"=timestamp(3493755753 s since 1904-01-01), "file name str"="D:\\Data\\Ultrasound\\LSCO\\LSCO22__130814c\\5_Cooling_2nd_try\\September_2014\\091614\\122.43100K_500_2500_2.10000V_0.00000T_Sep16-2014__19-42-33_001_091614.bin", "mod time(min)"=58229262.55, "file format"=enum."binary", "power(V)"=2.1, "Magn Field(T) "=0.0}, {"temperature"=122.165, "temperature str"="122.16500", "file path"=path "D:/Data/Ultrasound/LSCO/LSCO22__130814c/5_Cooling_2nd_try/September_2014/091614/122.16500K_500_2500_2.10000V_0.00000T_Sep16-2014__19-43-53_001_091614.bin", "last mod"=timestamp(3493755833 s since 1904-01-01), "file name str"="D:\\Data\\Ultrasound\\LSCO\\LSCO22__130814c\\5_Cooling_2nd_try\\September_2014\\091614\\122.16500K_500_2500_2.10000V_0.00000T_Sep16-2014__19-43-53_001_091614.bin", "mod time(min)"=58229263.88333333, "file format"=enum."binary", "power(V)"=2.1, "Magn Field(T) "=0.0}, {"temperature"=121.901, "temperature str"="121.90100", "file path"=path "D:/Data/Ultrasound/LSCO/LSCO22__130814c/5_Cooling_2nd_try/September_2014/091614/121.90100K_500_2500_2.10000V_0.00000T_Sep16-2014__19-45-12_001_091614.bin", "last mod"=timestamp(3493755912 s since 1904-01-01), "file name str"="D:\\Data\\Ultrasound\\LSCO\\LSCO22__130814c\\5_Cooling_2nd_try\\September_2014\\091614\\121.90100K_500_2500_2.10000V_0.00000T_Sep16-2014__19-45-12_001_091614.bin", "mod time(min)"=58229265.2, "file format"=enum."binary", "power(V)"=2.1, "Magn Field(T) "=0.0}, {"temperature"=121.649, "temperature str"="121.64900", "file path"=path "D:/Data/Ultrasound/LSCO/LSCO22__130814c/5_Cooling_2nd_try/September_2014/091614/121.64900K_500_2500_2.10000V_0.00000T_Sep16-2014__19-46-31_001_091614.bin", "last mod"=timestamp(3493755991 s since 1904-01-01), "file name str"="D:\\Data\\Ultrasound\\LSCO\\LSCO22__130814c\\5_Cooling_2nd_try\\September_2014\\091614\\121.64900K_500_2500_2.10000V_0.00000T_Sep16-2014__19-46-31_001_091614.bin", "mod time(min)"=58229266.516666666, "file format"=enum."binary", "power(V)"=2.1, "Magn Field(T) "=0.0}, {"temperature"=121.386, "temperature str"="121.38600", "file path"=path "D:/Data/Ultrasound/LSCO/LSCO22__130814c/5_Cooling_2nd_try/September_2014/091614/121.38600K_500_2500_2.10000V_0.00000T_Sep16-2014__19-47-51_001_091614.bin", "last mod"=timestamp(3493756071 s since 1904-01-01), "file name str"="D:\\Data\\Ultrasound\\LSCO\\LSCO22__130814c\\5_Cooling_2nd_try\\September_2014\\091614\\121.38600K_500_2500_2.10000V_0.00000T_Sep16-2014__19-47-51_001_091614.bin", "mod time(min)"=58229267.85, "file format"=enum."binary", "power(V)"=2.1, "Magn Field(T) "=0.0}, {"temperature"=121.132, "temperature str"="121.13200", "file path"=path "D:/Data/Ultrasound/LSCO/LSCO22__130814c/5_Cooling_2nd_try/September_2014/091614/121.13200K_500_2500_2.10000V_0.00000T_Sep16-2014__19-49-10_001_091614.bin", "last mod"=timestamp(3493756150 s since 1904-01-01), "file name str"="D:\\Data\\Ultrasound\\LSCO\\LSCO22__130814c\\5_Cooling_2nd_try\\September_2014\\091614\\121.13200K_500_2500_2.10000V_0.00000T_Sep16-2014__19-49-10_001_091614.bin", "mod time(min)"=58229269.166666664, "file format"=enum."binary", "power(V)"=2.1, "Magn Field(T) "=0.0}, {"temperature"=120.874, "temperature str"="120.87400", "file path"=path "D:/Data/Ultrasound/LSCO/LSCO22__130814c/5_Cooling_2nd_try/September_2014/091614/120.87400K_500_2500_2.10000V_0.00000T_Sep16-2014__19-50-30_001_091614.bin", "last mod"=timestamp(3493756230 s since 1904-01-01), "file name str"="D:\\Data\\Ultrasound\\LSCO\\LSCO22__130814c\\5_Cooling_2nd_try\\September_2014\\091614\\120.87400K_500_2500_2.10000V_0.00000T_Sep16-2014__19-50-30_001_091614.bin", "mod time(min)"=58229270.5, "file format"=enum."binary", "power(V)"=2.1, "Magn Field(T) "=0.0}, {"temperature"=120.614, "temperature str"="120.61400", "file path"=path "D:/Data/Ultrasound/LSCO/LSCO22__130814c/5_Cooling_2nd_try/September_2014/091614/120.61400K_500_2500_2.10000V_0.00000T_Sep16-2014__19-51-49_001_091614.bin", "last mod"=timestamp(3493756309 s since 1904-01-01), "file name str"="D:\\Data\\Ultrasound\\LSCO\\LSCO22__130814c\\5_Cooling_2nd_try\\September_2014\\091614\\120.61400K_500_2500_2.10000V_0.00000T_Sep16-2014__19-51-49_001_091614.bin", "mod time(min)"=58229271.81666667, "file format"=enum."binary", "power(V)"=2.1, "Magn Field(T) "=0.0}, {"temperature"=120.365, "temperature str"="120.36500", "file path"=path "D:/Data/Ultrasound/LSCO/LSCO22__130814c/5_Cooling_2nd_try/September_2014/091614/120.36500K_500_2500_2.10000V_0.00000T_Sep16-2014__19-53-08_001_091614.bin", "last mod"=timestamp(3493756388 s since 1904-01-01), "file name str"="D:\\Data\\Ultrasound\\LSCO\\LSCO22__130814c\\5_Cooling_2nd_try\\September_2014\\091614\\120.36500K_500_2500_2.10000V_0.00000T_Sep16-2014__19-53-08_001_091614.bin", "mod time(min)"=58229273.13333333, "file format"=enum."binary", "power(V)"=2.1, "Magn Field(T) "=0.0}, {"temperature"=120.108, "temperature str"="120.10800", "file path"=path "D:/Data/Ultrasound/LSCO/LSCO22__130814c/5_Cooling_2nd_try/September_2014/091614/120.10800K_500_2500_2.10000V_0.00000T_Sep16-2014__19-54-28_001_091614.bin", "last mod"=timestamp(3493756468 s since 1904-01-01), "file name str"="D:\\Data\\Ultrasound\\LSCO\\LSCO22__130814c\\5_Cooling_2nd_try\\September_2014\\091614\\120.10800K_500_2500_2.10000V_0.00000T_Sep16-2014__19-54-28_001_091614.bin", "mod time(min)"=58229274.46666667, "file format"=enum."binary", "power(V)"=2.1, "Magn Field(T) "=0.0}, {"temperature"=119.859, "temperature str"="119.85900", "file path"=path "D:/Data/Ultrasound/LSCO/LSCO22__130814c/5_Cooling_2nd_try/September_2014/091614/119.85900K_500_2500_2.10000V_0.00000T_Sep16-2014__19-55-47_001_091614.bin", "last mod"=timestamp(3493756547 s since 1904-01-01), "file name str"="D:\\Data\\Ultrasound\\LSCO\\LSCO22__130814c\\5_Cooling_2nd_try\\September_2014\\091614\\119.85900K_500_2500_2.10000V_0.00000T_Sep16-2014__19-55-47_001_091614.bin", "mod time(min)"=58229275.78333333, "file format"=enum."binary", "power(V)"=2.1, "Magn Field(T) "=0.0}, {"temperature"=119.604, "temperature str"="119.60400", "file path"=path "D:/Data/Ultrasound/LSCO/LSCO22__130814c/5_Cooling_2nd_try/September_2014/091614/119.60400K_500_2500_2.10000V_0.00000T_Sep16-2014__19-57-06_001_091614.bin", "last mod"=timestamp(3493756626 s since 1904-01-01), "file name str"="D:\\Data\\Ultrasound\\LSCO\\LSCO22__130814c\\5_Cooling_2nd_try\\September_2014\\091614\\119.60400K_500_2500_2.10000V_0.00000T_Sep16-2014__19-57-06_001_091614.bin", "mod time(min)"=58229277.1, "file format"=enum."binary", "power(V)"=2.1, "Magn Field(T) "=0.0}, {"temperature"=119.349, "temperature str"="119.34900", "file path"=path "D:/Data/Ultrasound/LSCO/LSCO22__130814c/5_Cooling_2nd_try/September_2014/091614/119.34900K_500_2500_2.10000V_0.00000T_Sep16-2014__19-58-26_001_091614.bin", "last mod"=timestamp(3493756706 s since 1904-01-01), "file name str"="D:\\Data\\Ultrasound\\LSCO\\LSCO22__130814c\\5_Cooling_2nd_try\\September_2014\\091614\\119.34900K_500_2500_2.10000V_0.00000T_Sep16-2014__19-58-26_001_091614.bin", "mod time(min)"=58229278.43333333, "file format"=enum."binary", "power(V)"=2.1, "Magn Field(T) "=0.0}, {"temperature"=119.104, "temperature str"="119.10400", "file path"=path "D:/Data/Ultrasound/LSCO/LSCO22__130814c/5_Cooling_2nd_try/September_2014/091614/119.10400K_500_2500_2.10000V_0.00000T_Sep16-2014__19-59-45_001_091614.bin", "last mod"=timestamp(3493756785 s since 1904-01-01), "file name str"="D:\\Data\\Ultrasound\\LSCO\\LSCO22__130814c\\5_Cooling_2nd_try\\September_2014\\091614\\119.10400K_500_2500_2.10000V_0.00000T_Sep16-2014__19-59-45_001_091614.bin", "mod time(min)"=58229279.75, "file format"=enum."binary", "power(V)"=2.1, "Magn Field(T) "=0.0}, {"temperature"=118.85, "temperature str"="118.85000", "file path"=path "D:/Data/Ultrasound/LSCO/LSCO22__130814c/5_Cooling_2nd_try/September_2014/091614/118.85000K_500_2500_2.10000V_0.00000T_Sep16-2014__20-01-05_001_091614.bin", "last mod"=timestamp(3493756865 s since 1904-01-01), "file name str"="D:\\Data\\Ultrasound\\LSCO\\LSCO22__130814c\\5_Cooling_2nd_try\\September_2014\\091614\\118.85000K_500_2500_2.10000V_0.00000T_Sep16-2014__20-01-05_001_091614.bin", "mod time(min)"=58229281.083333336, "file format"=enum."binary", "power(V)"=2.1, "Magn Field(T) "=0.0}, {"temperature"=118.609, "temperature str"="118.60900", "file path"=path "D:/Data/Ultrasound/LSCO/LSCO22__130814c/5_Cooling_2nd_try/September_2014/091614/118.60900K_500_2500_2.10000V_0.00000T_Sep16-2014__20-02-24_001_091614.bin", "last mod"=timestamp(3493756944 s since 1904-01-01), "file name str"="D:\\Data\\Ultrasound\\LSCO\\LSCO22__130814c\\5_Cooling_2nd_try\\September_2014\\091614\\118.60900K_500_2500_2.10000V_0.00000T_Sep16-2014__20-02-24_001_091614.bin", "mod time(min)"=58229282.4, "file format"=enum."binary", "power(V)"=2.1, "Magn Field(T) "=0.0}, {"temperature"=118.359, "temperature str"="118.35900", "file path"=path "D:/Data/Ultrasound/LSCO/LSCO22__130814c/5_Cooling_2nd_try/September_2014/091614/118.35900K_500_2500_2.10000V_0.00000T_Sep16-2014__20-03-43_001_091614.bin", "last mod"=timestamp(3493757023 s since 1904-01-01), "file name str"="D:\\Data\\Ultrasound\\LSCO\\LSCO22__130814c\\5_Cooling_2nd_try\\September_2014\\091614\\118.35900K_500_2500_2.10000V_0.00000T_Sep16-2014__20-03-43_001_091614.bin", "mod time(min)"=58229283.71666667, "file format"=enum."binary", "power(V)"=2.1, "Magn Field(T) "=0.0}, {"temperature"=118.111, "temperature str"="118.11100", "file path"=path "D:/Data/Ultrasound/LSCO/LSCO22__130814c/5_Cooling_2nd_try/September_2014/091614/118.11100K_500_2500_2.10000V_0.00000T_Sep16-2014__20-05-03_001_091614.bin", "last mod"=timestamp(3493757103 s since 1904-01-01), "file name str"="D:\\Data\\Ultrasound\\LSCO\\LSCO22__130814c\\5_Cooling_2nd_try\\September_2014\\091614\\118.11100K_500_2500_2.10000V_0.00000T_Sep16-2014__20-05-03_001_091614.bin", "mod time(min)"=58229285.05, "file format"=enum."binary", "power(V)"=2.1, "Magn Field(T) "=0.0}, {"temperature"=117.87, "temperature str"="117.87000", "file path"=path "D:/Data/Ultrasound/LSCO/LSCO22__130814c/5_Cooling_2nd_try/September_2014/091614/117.87000K_500_2500_2.10000V_0.00000T_Sep16-2014__20-06-22_001_091614.bin", "last mod"=timestamp(3493757182 s since 1904-01-01), "file name str"="D:\\Data\\Ultrasound\\LSCO\\LSCO22__130814c\\5_Cooling_2nd_try\\September_2014\\091614\\117.87000K_500_2500_2.10000V_0.00000T_Sep16-2014__20-06-22_001_091614.bin", "mod time(min)"=58229286.36666667, "file format"=enum."binary", "power(V)"=2.1, "Magn Field(T) "=0.0}, {"temperature"=117.621, "temperature str"="117.62100", "file path"=path "D:/Data/Ultrasound/LSCO/LS
